vi "ActionVIUI.vi"() -> ()   [LabVIEW 2015, in "ActionVI.lvclass"]
uses:
  ActionVI.lvclass
  <vilib>/NI/Configuration Framework/Node/NodeRef.ctl
  <vilib>/NI/Configuration Framework/Node/NISE_CEF_Node.lvclass
  <vilib>/NI/AMC/Message Queue.ctl
  <vilib>/NI/AMC/Message.ctl
  <vilib>/NI/Tools/Keyed Array/KeyedArray.ctl
  <vilib>/NI/Configuration Framework/Node/UserEventRef.ctl
  <vilib>/NI/Configuration Framework/Controls/EventCluster.ctl
  ActionVI.lvclass/ActionVI.ctl
  Read Action VI Properties.vi
  Write Action VI Properties.vi
  <vilib>/NI/AMC/Create Single Message.vi
  <vilib>/NI/AMC/Update Message Routing Info.vi
  <vilib>/NI/AMC/Send Message.vi
  <vilib>/NI/AMC/AMC.lvlib
  Configuration Tool.lvlib
  <vilib>/NI/Tools/Keyed Array/Tools_KeyedArray.lvlib
  <vilib>/NI/Configuration Framework/NISE_CEF_TreeControl.lvlib
panel:
  in  "Host Path to ActionVI":path
  in  "user event":T1
  in  "main queue":T2
  in  "node ref":T3
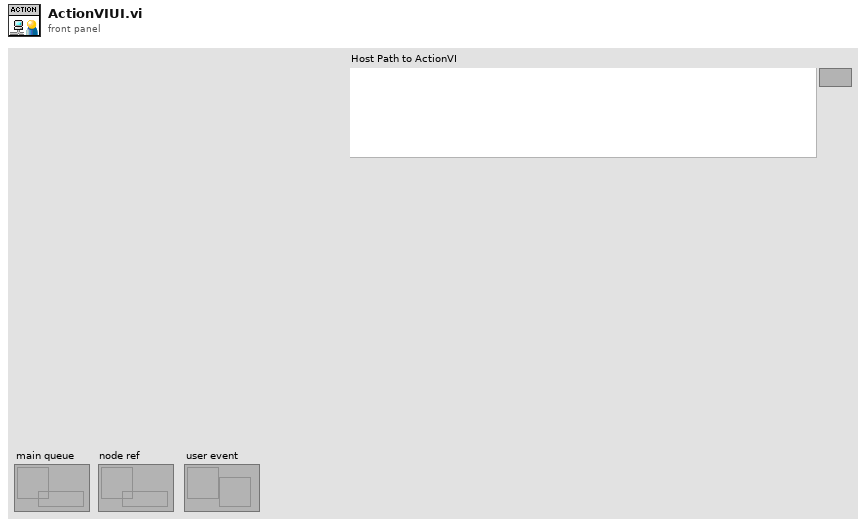
[diagram p1: front panel]
types:
  T1 = typedef "NISE_CEF_Node.lvclass/UserEventRef.ctl" = refnum<user-event>
  T2 = typedef "AMC.lvlib/Message Queue.ctl" = refnum<queue>
  T3 = typedef "NISE_CEF_Node.lvclass/NodeRef.ctl" = refnum<data-value>
  T4 = typedef "Path Cluster.ctl" = cluster{"Path":path, "Path Type":enum16{"Absolute", "To Base", "To Common Doc Dir", "To Application Data Dir"}}
  T5 = enum16{"Absolute", "To Base", "To Common Doc Dir", "To Application Data Dir"}
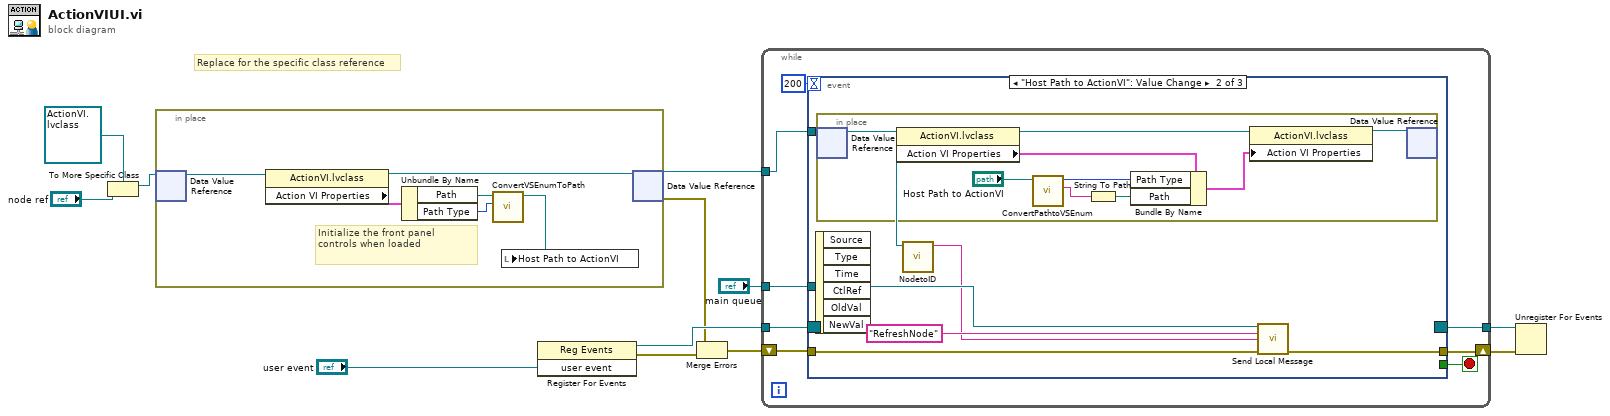
[diagram p0: block diagram]
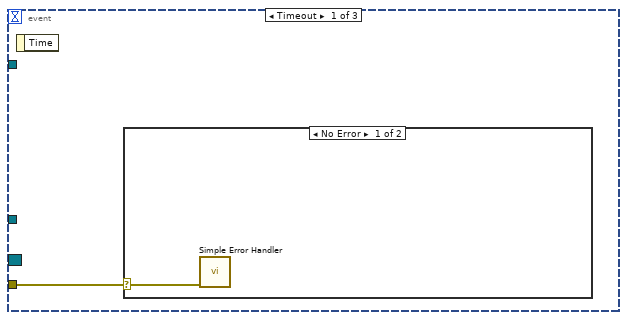
[diagram p2: hidden frame]
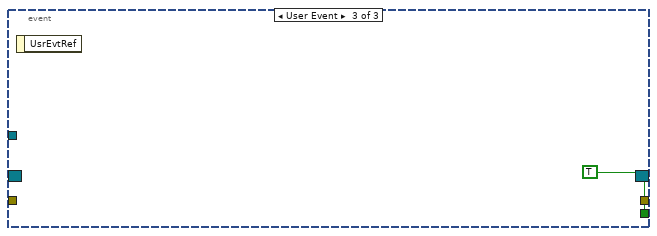
[diagram p4: hidden frame]
diagram:
  # "Replace for the specific class reference"
  n1 = To More Specific Class(target class=refnum<data-value> refnum ("data value reference"), reference="node ref") -> (specific class reference=w5:refnum<data-value>)  [unwired: 1 in, 1 out]
  n2 = in-place {
    # "Initialize the front panel controls when loaded"
    n3 = in-place-dvr #1(w5) -> (w18:refnum<class "ActionVI.lvclass">)  [unwired: 1 out]
    n4 = property class="ActionVI.lvclass"(reference=w18) -> (reference out=w17:refnum<class "ActionVI.lvclass">, "Action VI Properties"=w16:T4)  [unwired: 1 in, 1 out]
    n5 = Unbundle By Name(w16) -> ("Path"=w15:path, "Path Type"=w14:T5)
    n6 = call "ConvertVSEnumToPath.vi"("Source.Path Type"=w14, "Path In"=w15) -> ("appended path"=w13:path)  [unwired: 9 in]
    n7 = local write "Host Path to ActionVI"(w13) -> ()
    n8 = in-place-dvr #1(w17) -> (w12:refnum<data-value>, w2:errorcluster)
  }
  n9 = register-events("user event") -> (reference out=w9:refnum<event-registration>, error out=w3:errorcluster)  [unwired: 2 in]
  n10 = Merge Errors(w2, w3) -> (w1:errorcluster)
  n11 = while {
    tunnel: w12 -> [w26]
    tunnel: "main queue" -> [w25]
    tunnel: w9 -> [w23]
    tunnel: [w22] -> w8
    shift-right: [w20] -> w7
    shift-left: w1 -> [w19]
    stop <- w21 stop-if-true
    n12 = event shown="[1] \"Host Path to ActionVI\": Value Change" {
      selector: w23 -> [_ _ _]
      dyn-events: [_ _ _] -> w22
      timeout: 200 -> [_ _ _]
      tunnel: w26 -> [_ w32 _]
      tunnel: w25 -> [_ w33 _]
      tunnel: [_ _ TRUE] -> w21
      tunnel: [_ w30 _] -> w20
      tunnel: w19 -> [w27 w29 _]
      event Timeout {
        n13 = event-data() -> ()  [unwired: 1 in, 1 out]
        n14 = case shown="No Error" w27 {
          selector: w27 -> [w28 _]
          frame No Error {
            n15 = call <vilib>:"Simple Error Handler.vi"("error in (no error)"=w28) -> ()  [unwired: 4 in, 5 out]
          }
          frame Error {
          }
        }
      }
      event "Host Path to ActionVI": Value Change {
        n16 = event-data() -> ()  [unwired: 1 in, 6 out]
        n17 = in-place {
          n18 = in-place-dvr #2(w32) -> (w42:refnum<class "ActionVI.lvclass">)  [unwired: 1 out]
          n19 = property class="ActionVI.lvclass"(reference=w42) -> (reference out=w35:refnum<class "ActionVI.lvclass">, "Action VI Properties"=w41:T4)  [unwired: 1 in, 1 out]
          n20 = call "ConvertPathtoVSEnum.vi"("Path In"="Host Path to ActionVI") -> ("Remaining Path"=w39:string, "VS Enum Out"=w38:T5)  [unwired: 9 in]
          n21 = String To Path(string=w39) -> (path=w37:path)
          n22 = Bundle By Name(cluster=w41, "Path Type"=w38, "Path"=w37) -> (w40:T4)
          n23 = property class="ActionVI.lvclass"(reference=w35, "Action VI Properties"=w40) -> (reference out=w43:refnum<class "ActionVI.lvclass">)  [unwired: 1 in, 1 out]
          n24 = in-place-dvr #2(w43) -> ()  [unwired: 2 out]
        }
        n25 = call <vilib>:"NodetoID.vi"("node ref"=w32) -> ("ID"=w31:string)  [unwired: 9 in, 1 out]
        n26 = call <vilib>:"Send Local Message.vi"("message queue in"=w33, "message name"="RefreshNode" ("Message Name"), "message value"=w31, "error in"=w29) -> ("error out"=w30:errorcluster)  [unwired: 9 in, 2 out]
      }
      event User Event {
        n27 = event-data() -> ()  [unwired: 1 in, 1 out]
      }
    }
  }
  n28 = Unregister For Events(event registration refnum=w8, error in=w7) -> ()  [unwired: 1 out]
